vi "GetParameterCollectionConstraint.vi"(6 "ConstraintCategory":T5, 8 "error in (no error)":errorcluster, 9 "PicamValueType":T4=enum."Integer", 10 "PicamParameter":T6=15 items=["---Analog to Digital Conversion---"=1005, "AdcSpeed"=33, "AdcBitDepth"=34, "AdcAnalogGain"=35, "AdcQuality"=36, "AdcEMGain"=53, "CorrectPixelBias"=106, "---SENSOR LAYOUT---"=1000, "AcitveWidth"=1, "ActiveHeight"=2, "ActiveExtendedHeight"=160, "ActiveLeftMargin"=3, "ActiveTopMargin"=4, "ActiveRightMargin"=5, "ActiveBottomMargin"=6, "MaskedHeight"=7, "MaskedTopMargin"=8, "MaskedBottomMargin"=73, "SecondaryMaskedHeight"=75, "SecondaryActiveHeight"=76, "---READOUT CONTROL---"=1001, "ReadoutControlMode"=26, "ReadoutTimeCalculation"=27, "ReadoutPortCount"=28, "ReadoutOrientation"=54, "KineticsWindowHeight"=56, "SeNsRWindowHeight"=163, "VerticalShiftRate"=13, "Accumulations"=92, "EnableNondestructiveReadout"=128, "NondestructiveReadoutPeriod"=129, "---DATA ACQUISITION---"=1003, "Rois"=37, "NormalizeOrientation"=39, "DisableDataFormatting"=55, "ReadoutCount"=40, "ExactReadoutCountMaximum"=77, "FrameSize"=42, "FrameStride"=43, "FramesPerReadout"=44, "ReadoutStride"=45, "PixelBitDepth"=48, "TimeStampResolution"=69, "FrameTrackingBitDepth"=72, "---SENSOR TEMPERATURE---"=1002, "SensorTemperatureReading"=15], 11 "PicamHandle in":u64) -> (0 "error out":errorcluster, 2 "CollectionConstraint":T1, 3 "PicamHandle out":u64)   [LabVIEW 2019, in "PICam.lvlib"]
uses:
  PICam.lvlib
  Ctrls/PicamErrors.ctl
  types/PicamConstraintType.ctl
  types/CollectionConstraint.ctl
  types/ConstraintSeverity.ctl
  types/ConstraintScope.ctl
  Picam64.dll
  types/PicamParameter.ctl
  types/PicamConstraintCategory.ctl
  types/PicamValueType.ctl
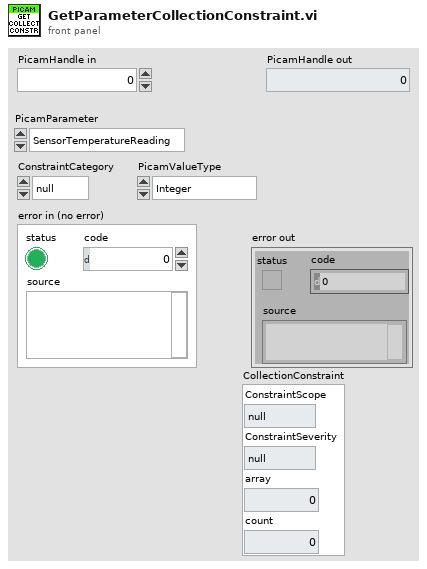
[diagram p1: front panel]
types:
  T1 = typedef "PICam.lvlib/CollectionConstraint.ctl" = cluster{"ConstraintScope":T2, "ConstraintSeverity":T3, "array":dbl, "count":i32}
  T2 = typedef "PICam.lvlib/ConstraintScope.ctl" = enum32{"null", "Independent", "Dependent"}
  T3 = typedef "PICam.lvlib/ConstraintSeverity.ctl" = enum32{"null", "Error", "Warning"}
  T4 = typedef "PICam.lvlib/PicamValueType.ctl" = enum32{"null", "Integer", "FloatingPoint", "Boolean", "Enumeration", "Rois", "LargeInteger", "Pulse", "Modulations"}
  T5 = typedef "PICam.lvlib/PicamConstraintCategory.ctl" = enum32{"null", "Capable", "Required", "Recommended"}
  T6 = typedef "PICam.lvlib/PicamParameter.ctl" = u32
  T7 = typedef "PICam.lvlib/PicamConstraintType.ctl" = enum32{"null", "None", "Range", "Collection", "Rois", "Pulse", "Modulations"}
  T8 = typedef "PICam.lvlib/PicamErrors.ctl" = i32
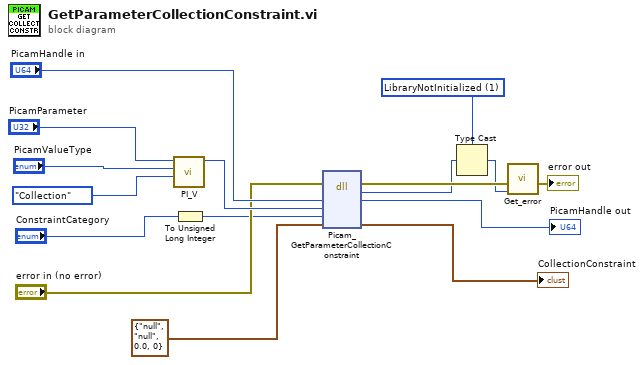
[diagram p0: block diagram]
diagram:
  w13 = T8 1 items=["LibraryNotInitialized"=1, "InvalidParameterValue"=2, "UnexpectedNullPointer"=3, "UnexpectedError"=4, "LibraryAlreadyInitialized"=5, "InvalidDemoModel"=6, "CameraAlreadyOpened"=7, "InvalidCameraID"=8, "InvalidHandle"=9, "ParameterValueIsReadOnly"=10, "ParameterHasInvalidValueType"=11, "ParameterDoesNotExist"=12, "ParameterHasInvalidConstraintType"=13, "ParameterValueIsIrrelevant"=14, "DeviceCommunicationFailed"=15, "InvalidEnumeratedType"=16, "EnumerationValueNotDefined"=17, "NotDiscoveringCameras"=18, "AlreadyDiscoveringCameras"=19, "AcquisitionInProgress"=20, "InvalidDemoSerialNumber"=21, "DemoAlreadyConnected"=22, "DeviceDisconnected"=23, "DeviceOpenElsewhere"=24, "ParameterIsNotOnlineable"=25, "ParameterIsNotReadable"=26, "AcquisitionNotInProgress"=27, "InvalidParameterValues"=28, "ParametersNotCommitted"=29, "InvalidAcquisitionBuffer"=30, "InsufficientMemory"=31, "TimeOutOccurred"=32, "AcquisitionUpdatedHandlerRegistered"=33, "NoCamerasAvailable"=34, "InvalidPointer"=35, "InvalidReadoutCount"=36, "InvalidReadoutTimeOut"=37, "InvalidConstraintCategory"=38, "InvalidCount"=39, "DemoNotSupported"=40, "NondestructiveReadoutEnabled"=41, "InvalidOperation"=42, "OperationCanceled"=43, "InvalidAcquisitionState"=44, "NoAccessoriesAvailable"=45, "AccessoryAlreadyOpened"=46, "InvalidAccessoryID"=47, "NotDiscoveringAccessories"=48, "AlreadyDiscoveringAccessories"=49, "ParameterIsNotWaitableStatus"=50, "InvalidWaitableStatusParameterTimeOut"=51, "ShutterOverheated"=52, "CameraFaulted"=53, "CenterWavelengthFaulted"=54] ("PICam_Error")
  n1 = call "PI_V.vi"("PicamConstraintType"=PicamConstraintType."Collection", "PicamValueType"="PicamValueType", "Numeric"="PicamParameter") -> ("PicamParameter value"=w8:u32)  [unwired: 8 in]
  n2 = To Unsigned Long Integer(number="ConstraintCategory") -> (unsigned 32bit integer=w3:u32)
  n3 = dll-call lib="Picam*.*" fn="Picam_GetParameterCollectionConstraint"(error in="error in (no error)", "PicamHandle"="PicamHandle in", "PicamParameter"=w8, "ConstraintCategory"=w3, "CollectionConstraint"=T1 {"ConstraintScope"=enum."null", "ConstraintSeverity"=enum."null", "array"=0.0, "count"=0}) -> (error out=w16:errorcluster, "error"=w15:i32, "PicamHandle"=→"PicamHandle out":u64, "CollectionConstraint"=→"CollectionConstraint":T1)  [unwired: 4 in, 1 out]
  n4 = Type Cast(type=w13, x=w15) -> (*(type *) &x=w14:T8)
  n5 = call "Get_error.vi"("PICam_Error"=w14, "error in (no error)"=w16) -> ("error out"=→"error out":errorcluster)  [unwired: 9 in]
